vi "Decompose LabVIEW Object.vi"(8 "error in (no error)":errorcluster, 11 "LabVIEW Object":refnum<class>) -> (0 "error out":errorcluster, 1 "Class Names":string[](array[string]), 2 "Library Versions":T1(array[cluster]), 3 "Private Data Clusters":variant[](array[variant]))   [LabVIEW 2017, in "Composition.lvlib"]
doc: "Decomposes a LabVIEW Object into its private data clusters from oldest ancestor to last decendant (same order as in Probe Watch Window)."
uses:
  Composition.lvlib
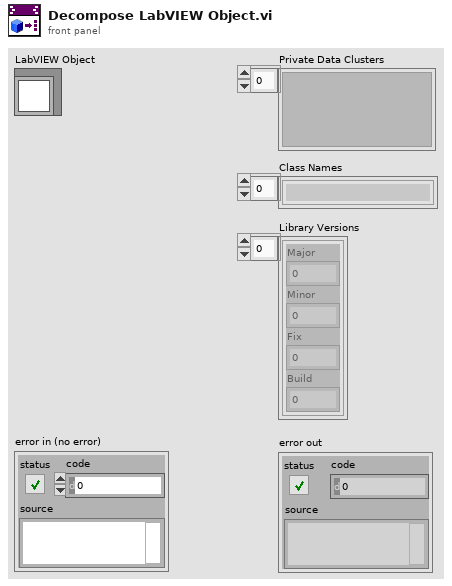
[diagram p1: front panel]
types:
  T1 = cluster{"Major":u16, "Minor":u16, "Fix":u16, "Build":u16}[]
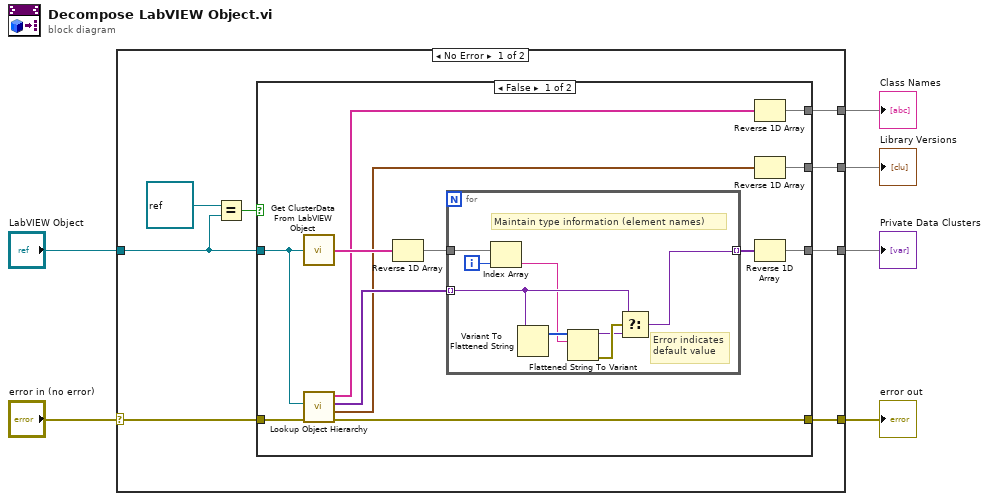
[diagram p0: block diagram]
diagram:
  n1 = case shown="No Error" "error in (no error)" {
    selector: "error in (no error)" -> [w11 w36]
    tunnel: [w14 _] -> w4
    tunnel: "LabVIEW Object" -> [w9 _]
    tunnel: [w10 w36] -> w3
    tunnel: [w13 _] -> w2
    tunnel: [w12 _] -> w1
    frame No Error {
      n2 = Equal?(x=refnum<class> refnum ("LabVIEW Object"), y=w9) -> (x = y?=w8:bool)
      n3 = case shown="False" w8 {
        tunnel: [w21 _] -> w14
        tunnel: w9 -> [w23 _]
        tunnel: [w18 _] -> w13
        tunnel: [w17 _] -> w12
        tunnel: w11 -> [w16 w35]
        tunnel: [w15 w35] -> w10
        frame False {
          n4 = call "Get ClusterData From LabVIEW Object.vi"("LabVIEW Object"=w23) -> ("Flattened Cluster Data"=w25:string[])
          n5 = call "Lookup Object Hierarchy.vi"("error in (no error)"=w16, "LabVIEW Object"=w23) -> ("error out"=w15:errorcluster, "Library Versions"=w19:T1, "Private Data Clusters"=w22:variant[], "Class Names"=w20:string[])  [unwired: 6 in]
          n6 = Reverse 1D Array(array=w25) -> (reversed array=w26:string[])
          n7 = for {
            tunnel: w26 -> [w30]
            tunnel: [w27] -> w24 mode=indexing
            tunnel: w22 -> [w31] mode=indexing
            i -> [w29]
            # "Error indicates\ndefault value"
            # "Maintain type information (element names)"
            n8 = Index Array(array=w30, index=w29) -> (element=w28:string)
            n9 = Variant To Flattened String(Variant=w31) -> (1:w34:i16[])  [unwired: 1 out]
            n10 = Flattened String To Variant(6:w28, 7:w34) -> (0:w33:errorcluster, 3:w32:variant)  [unwired: 1 in]
            n11 = Select(t=w31, s=w33, f=w32) -> (s? t:f=w27:variant)
          }
          n12 = Reverse 1D Array(array=w20) -> (reversed array=w18:string[])
          n13 = Reverse 1D Array(array=w19) -> (reversed array=w17:T1)
          n14 = Reverse 1D Array(array=w24) -> (reversed array=w21:variant[])
        }
        frame True {
          # "Ignore LabVIEW Object (mother of all objects in LV)"
        }
      }
    }
    frame Error {
    }
  }
  "Private Data Clusters" <- w4
  "error out" <- w3
  "Class Names" <- w2
  "Library Versions" <- w1
